vi "Z Scale Update.vi"(6 "Control Ref Queue":T1, 8 "error in (no error)":errorcluster, 9 "Kind":enum16{"X-Scale", "Y-Scale", "Z-Scale"}(ring), 10 "NewRange":T2, 11 "2D Plot.lvclass in":refnum<class "2D Compass.lvclass">) -> (0 "error out":errorcluster, 3 "2D Plot.lvclass out":refnum<class "2D Compass.lvclass">)   [LabVIEW 2017, in "2D Compass.lvclass"]
uses:
  <vilib>/Math Plots/2D Math Plots/2D Compass/2D Compass/2D Compass.lvclass
  e:/builds/penguin/labview/branches/2017/dev/dist/vi.lib/Math Plots/2D Math Plots/2D Plot/2D Plot/2D Plot.lvclass
  <vilib>/Utility/miscctls.llb/LVRangeTypeDef.ctl
  <vilib>/Math Plots/2D Math Plots/2D Plot/Action String/2DMathPlot Ctrl Act Queue.ctl
  <vilib>/Math Plots/2D Math Plots/2D Plot/Action String/2DMathPlot Ctrl Act Cluster.ctl
  <vilib>/Math Plots/2D Math Plots/2D Plot/Action String/2DMathPlot State Class.ctl
  <vilib>/Math Plots/2D Math Plots/2D Plot/2D Plot/2D Plot.lvclass
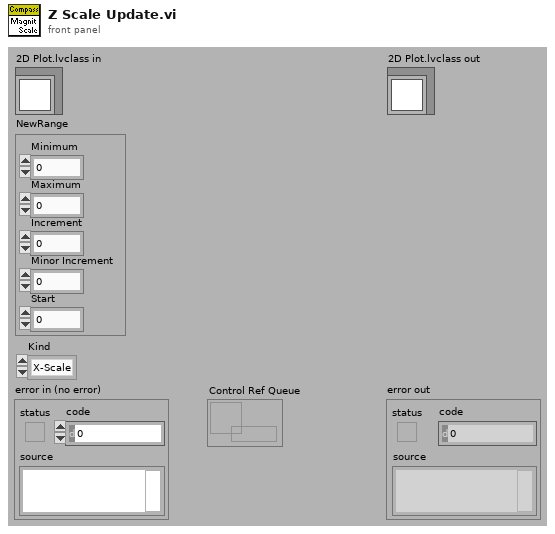
[diagram p1: front panel]
types:
  T1 = typedef "2DMathPlot Ctrl Act Queue.ctl" = refnum<queue>
  T2 = typedef "LVRangeTypeDef.ctl" = cluster{"Minimum":dbl, "Maximum":dbl, "Increment":dbl, "Minor Increment":dbl, "Start":dbl}
  T3 = typedef "2DMathPlot Ctrl Act Cluster.ctl" = cluster{"Plot Area Ref":refnum<vi>, "Z Axis Ref":refnum<vi>, "Legend Ref":refnum<vi>, "XControl Ref":refnum<vi>, "Facade Ref":refnum<vi>, "Display State Change Class":T4}
  T4 = typedef "2DMathPlot State Class.ctl" = enum16{"Update All (Undo)", "Update General", "Update Appearance", "Update Format", "Update Scale", "Update Marker", "Update Cursor", "None"}
  T5 = typedef "2D Plot.lvclass/Property Cluster.ctl" = cluster{"Graph General":T6, "Format Property":string[], "Scale Array":T7, "Cursor Property":T10, "Annotation List":T12, "Active Cursor":i32, "Active Plot":i32}
  T6 = typedef "2D Plot.lvclass/Graph General Property.ctl" = cluster{"Palette Visible":cluster{"Graph Legend":bool, "Plot Legend":bool, "Auto size":bool, "Number of Plots":u32, "X Scrollbar":bool, "Scale Legend":bool, "Cursor Legend":bool}, "Plot Area Color":cluster{"FG Color":u32, "BG Color":u32}, "Bounds Size":cluster{"Width":u32, "Height":u32}, "Plot Area Bounds":cluster{"Left":i16, "Top":i16, "Right":i16, "Bottom":i16}}
  T7 = typedef "2D Plot.lvclass/Scale Array.ctl" = T8[]
  T8 = typedef "2D Plot.lvclass/Scale Cluster.ctl" = cluster{"General":cluster{"Editable":bool, "Flipped":bool, "Mapping Mode":u8, "Visible":bool, "Style":u8, "Scale Fit":u8}, "Offset and Multiplier":T9, "Range":cluster{"Minimum":dbl, "Maximum":dbl, "Increment":dbl, "Minor Increment":dbl, "Start":dbl}, "Tick Color":cluster{"Major Color":u32, "Minor Color":u32}, "Gird Color":cluster{"Major Color":u32, "Minor Color":u32}, "Marker":cluster{"Visible":bool, "FG Color":u32, "BG Color":u32, "Font Name":string, "Font Size":u32, "Font Bold":bool, "Font Italic":bool, "Font Strikeout":bool, "Font Underline":bool}, "Name Label":cluster{"Visible":bool, "FG Color":u32, "BG Color":u32, "Font Name":string, "Font Size":u32, "Font Bold":bool, "Font Italic":bool, "Font Strikeout":bool, "Font Underline":bool, "Justification":enum16{"Left", "Center", "Right"}, "Text":string}}
  T9 = typedef "LVOffsetAndMultiplierTypeDef.ctl" = cluster{"Offset":dbl, "Multiplier":dbl}
  T10 = typedef "2D Plot.lvclass/Cursor Property.ctl" = cluster{"Cursor List":T11, "Cursor List Addtional":cluster{"Cursor Selection Color":u32, "Line Style":u8, "Line Width":u8, "Visible":bool}[]}
  T11 = typedef "LVCursorListTypeDef.ctl" = cluster{"Name":string, "Color":u32, "Style":u8, "Point Style":u8, "Name Visible":bool, "Allow Drag":bool, "Cursor Mode":u32, "Plot":i32, "Index":i32, "Position":cluster{"X":dbl, "Y":dbl}, "X Scale":u32, "Y Scale":u32, "Watch Plots":i32[], "Watch All Plots":bool, "Plot Area":i32, "Label Offset":cluster{"X":dbl, "Y":dbl}}[]
  T12 = typedef "LVAnnotationListTypeDef.ctl" = cluster{"Name":string, "Color":u32, "Style":u8, "Point Style":u8, "Name Visible":bool, "Allow Drag":bool, "Annotation Mode":u32, "Plot":i32, "Index":i32, "Position":cluster{"X":dbl, "Y":dbl}, "X Scale":u32, "Y Scale":u32, "Show Arrow":bool, "Lock Name":bool, "Plot Area":i32, "Label Offset":cluster{"X":dbl, "Y":dbl}}[]
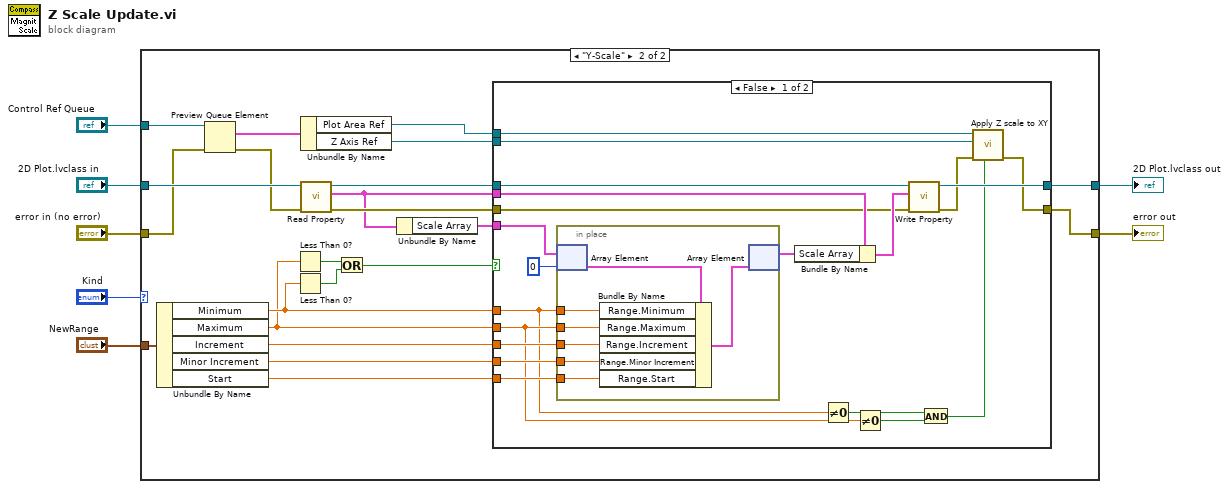
[diagram p0: block diagram]
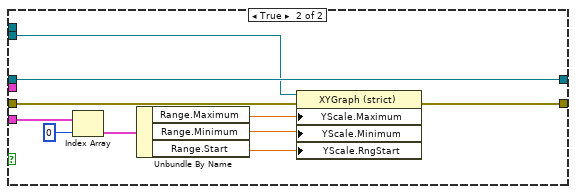
[diagram p3: hidden frame]
diagram:
  n1 = case shown="\"Y-Scale\"" "Kind" {
    tunnel: "Control Ref Queue" -> [_ w16]
    tunnel: [w8 w11] -> w6
    tunnel: "2D Plot.lvclass in" -> [w9 w21]
    tunnel: [w9 w31] -> w4
    tunnel: "NewRange" -> [_ w27]
    tunnel: "error in (no error)" -> [w8 w13]
    frame "X-Scale", Default {
    }
    frame "Y-Scale" {
      n2 = Unbundle By Name(w27) -> ("Minimum"=w26:dbl, "Maximum"=w25:dbl, "Increment"=w28:dbl, "Minor Increment"=w29:dbl, "Start"=w30:dbl)
      n3 = Preview Queue Element(queue=w16, error in (no error)=w13) -> (element=w15:T3, error out=w12:errorcluster)  [unwired: 3 out]
      n4 = Less Than 0?(x=w25) -> (x < 0?=w24:bool)
      n5 = Less Than 0?(x=w26) -> (x < 0?=w23:bool)
      n6 = Unbundle By Name(w15) -> ("Plot Area Ref"=w10:refnum<vi>, "Z Axis Ref"=w14:refnum<vi>)
      n7 = call <vilib>:"Read Property.vi"("error in (no error)"=w12, "2D Plot.lvclass in"=w21) -> ("error out"=w19:errorcluster, "XY Graph Property Cluster"=w17:T5, "2D Plot.lvclass out"=w20:refnum<class "2D Compass.lvclass">)  [unwired: 7 in]
      n8 = Or(x=w24, y=w23) -> (x .or. y?=w22:bool)
      n9 = Unbundle By Name(w17) -> ("Scale Array"=w18:T7)
      n10 = case shown="False" w22 {
        tunnel: w20 -> [w43 w68]
        tunnel: [w51 w68] -> w31
        tunnel: w30 -> [w49 _]
        tunnel: w29 -> [w48 _]
        tunnel: w28 -> [w47 _]
        tunnel: w19 -> [w42 w61]
        tunnel: [w37 w60] -> w11
        tunnel: w26 -> [w35 _]
        tunnel: w25 -> [w36 _]
        tunnel: w17 -> [w44 _]
        tunnel: w18 -> [w41 w67]
        tunnel: w14 -> [w40 w59]
        tunnel: w10 -> [w39 _]
        frame False {
          n11 = in-place {
            in-place-border: w35 -> [w56]
            in-place-border: w36 -> [w55]
            in-place-border: w47 -> [w54]
            in-place-border: w48 -> [w53]
            in-place-border: w49 -> [w52]
            n12 = in-place-array #1(w41, 0) -> (w58:T8)
            n13 = Bundle By Name(cluster=w58, "Range.Minimum"=w56, "Range.Maximum"=w55, "Range.Increment"=w54, "Range.Minor Increment"=w53, "Range.Start"=w52) -> (w57:T8)
            n14 = in-place-array #1(w57) -> (w45:T7)  [unwired: 1 out]
          }
          n15 = Bundle By Name(cluster=w44, "Scale Array"=w45) -> (w50:T5)
          n16 = Not Equal To 0?(x=w35) -> (x != 0?=w33:bool)
          n17 = Not Equal To 0?(x=w36) -> (x != 0?=w34:bool)
          n18 = call <vilib>:"Write Property.vi"("error in (no error)"=w42, "XY Graph Property Cluster"=w50, "2D Plot.lvclass in"=w43) -> ("error out"=w38:errorcluster, "2D Plot.lvclass out"=w51:refnum<class "2D Compass.lvclass">)  [unwired: 7 in]
          n19 = And(x=w33, y=w34) -> (x .and. y?=w32:bool)
          n20 = call <vilib>:"Apply Z scale to XY.vi"("Enlarge Z scale?"=w32, "error in (no error)"=w38, "Z Axis Ref"=w40, "Plot Area Ref"=w39) -> ("error out"=w37:errorcluster)  [unwired: 7 out]
        }
        frame True {
          n21 = Index Array(array=w67, index=0) -> (element=w65:T8)
          n22 = Unbundle By Name(w65) -> ("Range.Maximum"=w62:dbl, "Range.Minimum"=w63:dbl, "Range.Start"=w64:dbl)
          n23 = property class="XYGraph (strict)"(reference=w59, error in=w61, "YScale.Maximum"=w62, "YScale.Minimum"=w63, "YScale.RngStart"=w64) -> (error out=w60:errorcluster)  [unwired: 1 out]
        }
      }
    }
  }
  "2D Plot.lvclass out" <- w4
  "error out" <- w6
